vi "ProgressBar.vi"(6 "stop":bool, 9 "Current":i32, 10 "High":i32, 11 "Message":string) -> ()   [LabVIEW 2017]
doc: "10/01/2010\n\nNational Analytics (TLE)\n\nProgress bar VI. This should remain modal."
panel:
  in  "Abort":bool
  out "Progress":i32(slide) max=32 scale=0.0..3.0
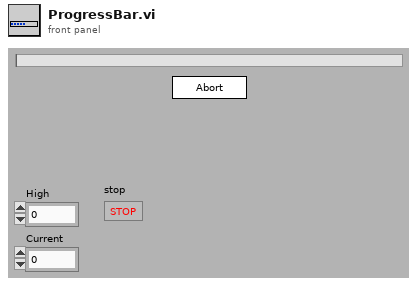
[diagram p1: front panel]
types:
  T1 = enum32{"Invalid", "Standard", "Closed", "Hidden", "Minimized", "Maximized"}
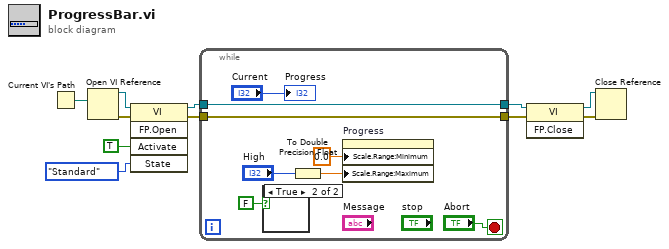
[diagram p0: block diagram]
diagram:
  n1 = Current VI's Path() -> (path=w9:path)
  n2 = Open VI Reference(vi path=w9) -> (vi reference=w11:refnum<vi>, error out=w10:errorcluster)  [unwired: 5 in]
  n3 = invoke class="VI" method="FP.Open"(reference=w11, error in=w10, "Activate"=TRUE ("Activate?"), "State"=T1."Standard") -> (reference out=w8:refnum<vi>, error out=w6:errorcluster)  [unwired: 1 in, 3 out]
  n4 = while {
    tunnel: [w16] -> w7
    tunnel: w8 -> [w16]
    tunnel: w6 -> [w15]
    tunnel: [w15] -> w5
    stop <- "Abort" stop-if-true
    n5 = case shown="True" FALSE {
      frame False {
      }
      frame True {
      }
    }
    n6 = To Double Precision Float(number="High") -> (double precision float=w17:dbl)
    n7 = property on="Progress" class="Slide (strict)"("Scale.Range:Minimum"=0.0, "Scale.Range:Maximum"=w17) -> ()  [unwired: 2 in, 2 out]
    "Progress" <- "Current"
  }
  n8 = invoke class="VI" method="FP.Close"(reference=w7, error in=w5) -> (reference out=w4:refnum<vi>, error out=w3:errorcluster)  [unwired: 1 in, 1 out]
  n9 = Close Reference(reference=w4, error in (no error)=w3) -> ()  [unwired: 1 out]
